vi "lsl push chunk str.vi"(8 "error in (no error)":errorcluster, 9 "data_elements":u32, 10 "data":string, 11 "out":cluster{}) -> (0 "error out":errorcluster, 2 "function return":i32, 3 "out out":cluster{})   [LabVIEW 2018, in "liblsl-LabVIEW.lvlib"]
doc: "extern LIBLSL_C_API int32_t lsl_push_chunk_str(lsl_outlet out, const char **data, unsigned long data_elements);"
uses:
  <userlib>/liblsl-LabVIEW/liblsl-LabVIEW.lvlib
  <userlib>/liblsl-LabVIEW/liblsl64.dll
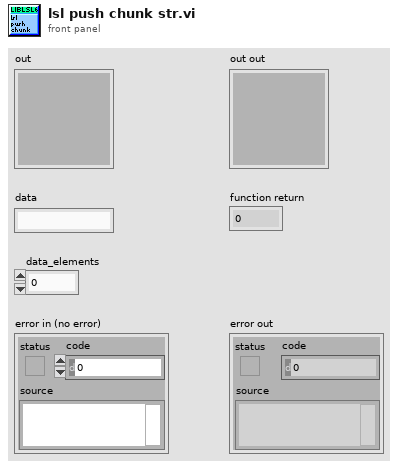
[diagram p1: front panel]
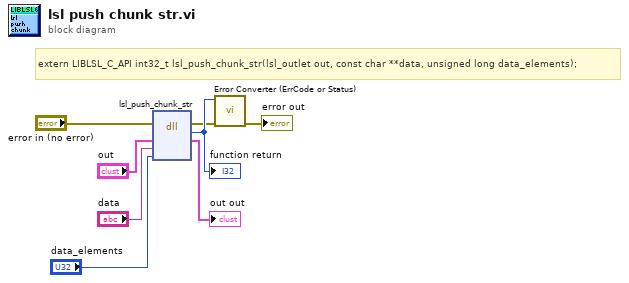
[diagram p0: block diagram]
diagram:
  # "extern LIBLSL_C_API int32_t lsl_push_chunk_str(lsl_outlet out, const char **data, unsigned long data_elements);"
  n1 = dll-call lib="C:/Program Files/National Instruments/LabVIEW 2018/user.lib/liblsl-LabVIEW/liblsl64.*" fn="lsl_push_chunk_str"(error in="error in (no error)", "out"="out", "data"="data", "data_elements"="data_elements") -> (error out=w2:errorcluster, w8:i32, "out"=→"out out":cluster{})  [unwired: 4 in, 1 out]
  "function return" <- w8
  n2 = call <userlib>:"Error Converter (ErrCode or Status).vi"("error in (no error)"=w2, "error code"=w8) -> ("error out"=→"error out":errorcluster)  [unwired: 9 in]
